vi "11-1 hp 33120a - Waveform Config sol.vi"(4 "unit (Vpp:0)":u16(ring)=1 items=["Vpp", "Vrms", "dB"], 5 "offset (0.00 V)":dbl min=-10.0 max=10.0 format="%.2f", 6 "amplitude (1.0 Vrms)":dbl=1.0 min=0.05 max=20.0 format="%.2f", 7 "frequency (1000 Hz)":dbl=1000.0 min=0.01 max=15000000.0 format="%.2f", 8 "error in (no error)":errorcluster, 9 "duty cycle (50 %)":i32=50 min=20 max=80, 10 "waveform shape (sine:1)":T1(ring)=enum."Noise", 11 "VISA session":refnum<visa-resource-name>) -> (0 "error out":errorcluster)   [LabVIEW 2012]
doc: "Performs the basic waveform configuration.\n\nThe instrument must be initialized for this example to function properly."
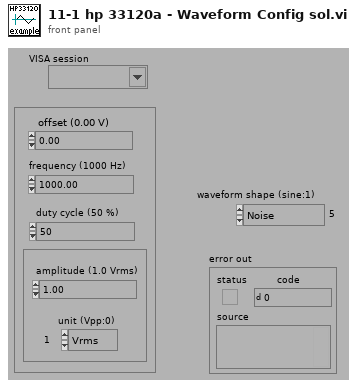
[diagram p1: front panel]
types:
  T1 = enum16{"DC", "Sine", "Square", "Triangle", "Ramp", "Noise", "Sinc", "Neg. Ramp", "Exp. Rise", "Exp. Fall", "Cardiac"}
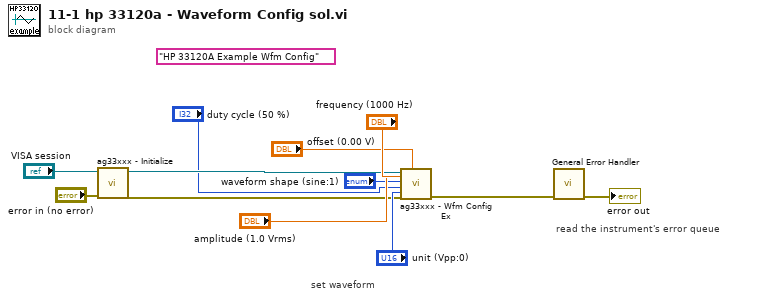
[diagram p0: block diagram]
diagram:
  (unwired) "HP 33120A Example Wfm Config"
  # "read the instrument's error queue"
  # "set waveform"
  n1 = call <instrlib>:"ag33xxx - Initialize.vi"("error in (no error)"="error in (no error)", "Instrument Resource Name"="VISA session") -> ("error out"=w3:errorcluster, "dup VISA session"=w6:refnum<visa-resource-name>)  [unwired: 8 in]
  n2 = call <instrlib>:"ag33xxx - Wfm Config Ex.vi"("Unit (0: Vpp)"="unit (Vpp:0)", "Offset (0.00 V)"="frequency (1000 Hz)", "Amplitude (0.1 Vpp)"="offset (0.00 V)", "Frequency (1000 Hz)"="amplitude (1.0 Vrms)", "error in (no error)"=w3, "Duty Cycle (50 %)"="duty cycle (50 %)", "Waveform Shape (1: Sine)"="waveform shape (sine:1)", "VISA session"=w6) -> ("error out"=w2:errorcluster)  [unwired: 3 in]
  n3 = call <vilib>:"General Error Handler.vi"("error in (no error)"=w2) -> ("error out"=→"error out":errorcluster)  [unwired: 10 in, 4 out]
